vi "GetSequenceSettings.vi"(0 "object in":refnum<class "Experiment2.lvclass">, 5 "error in (no error)":errorcluster) -> (14 "object out":refnum<class "Experiment2.lvclass">, 15 "Sequence Settings":T1={"Master Pulse Settings"={"Mode"=1, "Source"=1, "Interval"=1.0, "Burst"=0}, "Capture mode"=0, "Frames"=0, "Dcam Trigger Source"=1, "External Options"={"Polarity"=1, "Delay"=0.0}, "ExposureTime(ms)"=0.0} {"External Options"."Polarity" items=["Negative"=1, "Positive"=2]; "Dcam Trigger Source" items=["Internal"=1, "External"=2, "Software"=3, "Master Pulse"=4]; "Capture mode" items=["Snap", "Sequence"]; "Master Pulse Settings"."Source" items=["External"=1, "Software"=2]; "Master Pulse Settings"."Mode" items=["Continuous"=1, "Start"=2, "Burst"=3]}, 19 "error out":errorcluster)   [LabVIEW 2021, in "Experiment2.lvclass"]
uses:
  Experiment2.lvclass
  Experiment2.lvclass/Experiment2.ctl
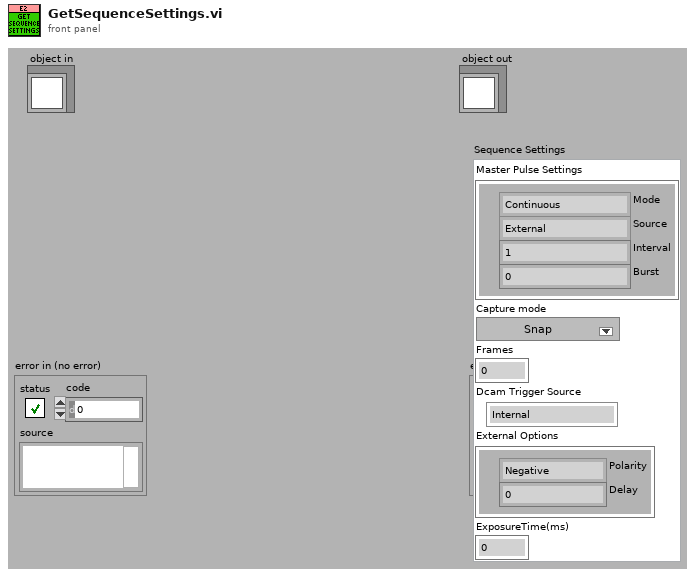
[diagram p1: front panel]
types:
  T1 = cluster{"Master Pulse Settings":cluster{"Mode":u32, "Source":u32, "Interval":dbl, "Burst":u32}, "Capture mode":i32, "Frames":i32, "Dcam Trigger Source":i32, "External Options":cluster{"Polarity":i32, "Delay":dbl}, "ExposureTime(ms)":dbl}
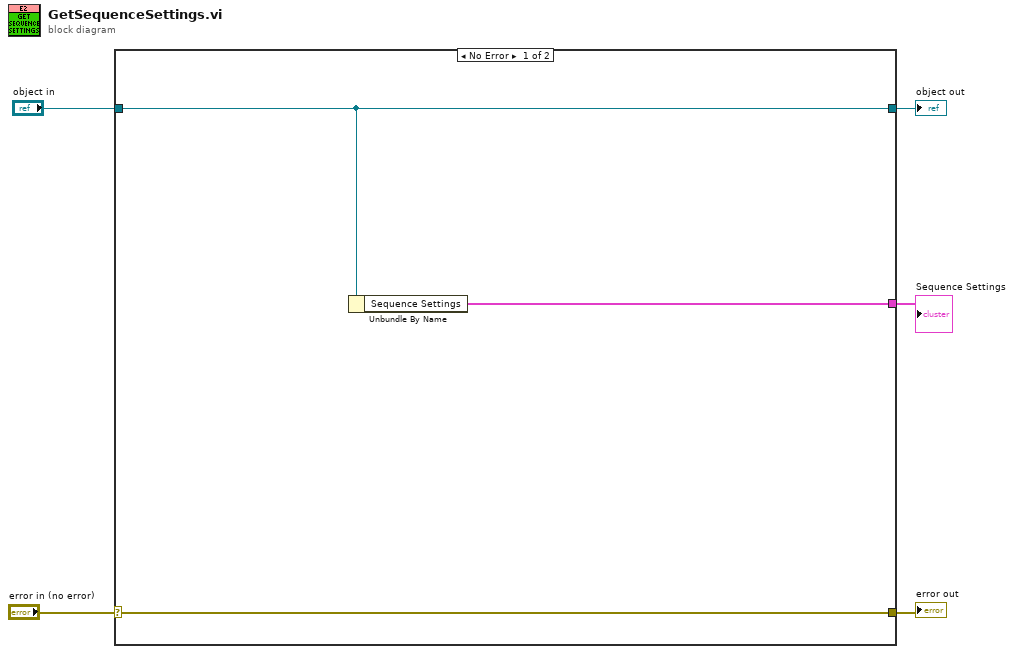
[diagram p0: block diagram]
diagram:
  n1 = case shown="No Error" "error in (no error)" {
    selector: "error in (no error)" -> [w7 w10]
    tunnel: [w7 w10] -> w4
    tunnel: [w6 w9] -> w2
    tunnel: "object in" -> [w6 w9]
    tunnel: [w8 _] -> w1
    frame No Error {
      n2 = Unbundle By Name(w6) -> ("Sequence Settings"=w8:T1)
    }
    frame Error {
    }
  }
  "error out" <- w4
  "object out" <- w2
  "Sequence Settings" <- w1
